vi "Sample changer.vi"() -> ()   [LabVIEW 2016, in "Top Level.lvlib"]
uses:
  Top Level.lvlib
  Sample Changer 2008 BETA 3.10.3/Visual Readback/half extended piston (push).ctl
  Sample Changer 2008 BETA 3.10.3/Visual Readback/half extended piston (push-in).ctl
  Sample Changer 2008 BETA 3.10.3/Visual Readback/Sample Rod (mid).ctl
  Sample Changer 2008 BETA 3.10.3/Visual Readback/Sample Rod (up-empty).ctl
  Sample Changer 2008 BETA 3.10.3/Visual Readback/Sample Rod (up-cathode).ctl
  Sample Changer 2008 BETA 3.10.3/Visual Readback/Sample Rod (down).ctl
  Sample Changer 2008 BETA 3.10.3/Visual Readback/Error - 2 Cathodes in the Rod.ctl
  Sample Changer 2008 BETA 3.10.3/Visual Readback/Wheel Gate Valve.ctl
panel:
  out "Wheel Gate Valve":T1
  out "Error - 2 Cathodes In Wheel":T2
  out "Error - 2 Cathodes In Rod":T2
  out "Sample Rod (down)":T3
  out "Wheel (Rod through)":bool
  out "Wheel (Empty)":bool
  out "Wheel (non-cathode position)":bool
  out "Wheel (cathode position)":bool
  out "Sample Rod (up-cathode)":T4
  out "Sample Rod (empty)":T5
  out "Sample Rod (mid)":T6
  out "half extended piston (in)":T7
  out "Extended Piston (in)":bool
  out "half extended piston (out)":T8
  out "Extended Piston (out)":bool
  in  "Encoder Home Off-Set":dbl=2790.0
  in  "sample number 2":i16
  out "Shared Network Variable Error":errorcluster
  out "Bellows Pressure String Read Error":errorcluster
  out "Source Pressure String Read Error":errorcluster
  out "output 1":dbl
  out "output 2":dbl
  in  "vent system":bool
  in  "stop":bool
  out "change sample":bool
  in  "cold cathode":dbl format="%#_3e"
  in  "Bellows pressure(torr)":string
  in  "Source pressure(torr)":string
  out "read position":dbl
  out "insert in":bool
  out "insert out":bool
  out "retract in":bool
  out "retract out":bool
  out "rod  down":bool
  out "rod up":bool
  out "sc gv closed":bool
  out "sc gv open":bool
  in  "rotate wheel":bool
  in  "sample number":i16
  in  "sc control":string
  in  "turn cold cathode off":bool
  in  "turn cold cathode on":bool
  in  "insert in":bool
  in  "insert out":bool
  in  "pump out system":bool
  in  "retract in":bool
  in  "retract out":bool
  in  "rod down":bool
  in  "rod up":bool
  in  "chamber valve close":bool
  in  "chamber valve open":bool
  # "Opens or Closes Wheel chamber valve"
  # "rotate wheel or change sample"
  # "Inserts sample into wheel"
  # "Pushes sample out of wheel"
  # "Raises or lowers Sample Rod"
  # "Turn cold cathode gauge on and off"
  # "If the cathode position is too low:\nYou have to increase the value.\nToo high, you have to lower it."
  # "vent system= isolate wheel chamber from bellows and source\nPump out system = re-connect wheel chamber to bellows and source"
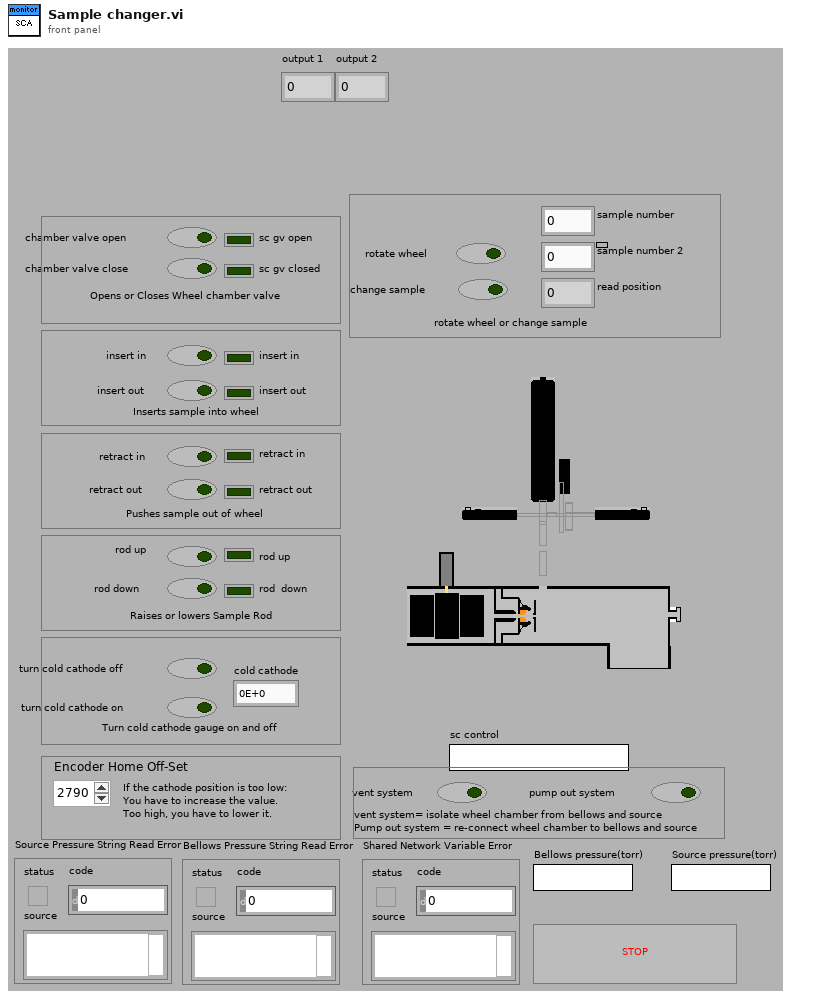
[diagram p1: front panel]
types:
  T1 = typedef "Wheel Gate Valve.ctl" = bool
  T2 = typedef "Error - 2 Cathodes in the Rod.ctl" = bool
  T3 = typedef "Sample Rod (down).ctl" = bool
  T4 = typedef "Sample Rod (up-cathode).ctl" = bool
  T5 = typedef "Sample Rod (up-empty).ctl" = bool
  T6 = typedef "Sample Rod (mid).ctl" = bool
  T7 = typedef "half extended piston (push-in).ctl" = bool
  T8 = typedef "half extended piston (push).ctl" = bool
  T9 = typedef "Device Position Enum.ctl" = enum16{"Unknown", "Actuator Is Moving", "Actuator Is Extended", "Actuator Is Retracted", "Disabled"}
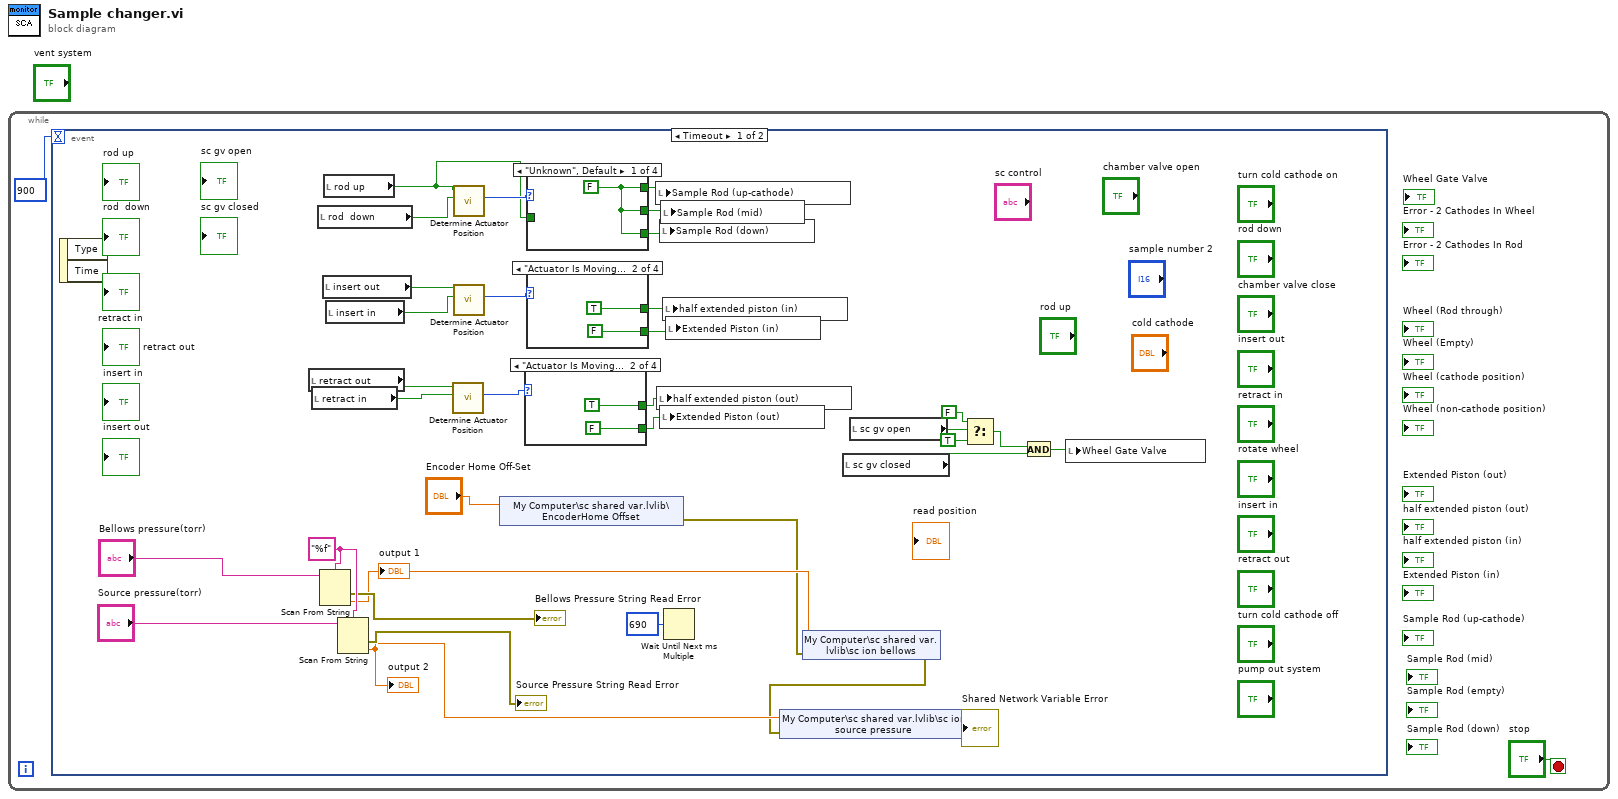
[diagram p0: block diagram]
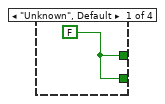
[diagram p2: hidden frame]
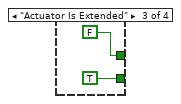
[diagram p3: hidden frame]
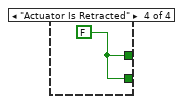
[diagram p4: hidden frame]
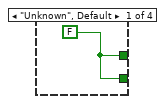
[diagram p5: hidden frame]
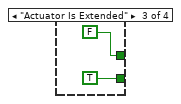
[diagram p6: hidden frame]
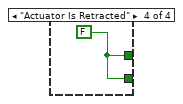
[diagram p7: hidden frame]
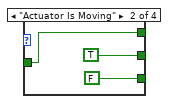
[diagram p8: hidden frame]
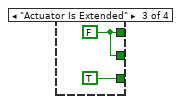
[diagram p9: hidden frame]
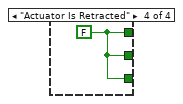
[diagram p10: hidden frame]
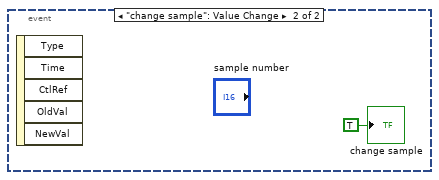
[diagram p11: hidden frame]
diagram:
  n1 = while {
    stop <- "stop" stop-if-true
    n2 = event shown="[0] Timeout" {
      selector: _ -> [_ _]
      dyn-events: _ -> [_ _]
      timeout: 900 -> [_ _]
      event Timeout {
        w35 = "%f" ("format string")
        n3 = event-data() -> ()  [unwired: 1 in, 2 out]
        n4 = local read "retract out"() -> (w5:bool)
        n5 = local read "retract in"() -> (w4:bool)
        n6 = local read "rod  down"() -> (w14:bool)
        n7 = Scan From String(format string=w35, input string="Bellows pressure(torr)") -> (error out=→"Bellows Pressure String Read Error":errorcluster, output 1=w32:dbl)  [unwired: 3 in, 2 out]
        "output 1" <- w32
        n8 = local read "insert out"() -> (w7:bool)
        n9 = local read "rod up"() -> (w3:bool)
        n10 = local read "insert in"() -> (w6:bool)
        n11 = Scan From String(format string=w35, input string="Source pressure(torr)") -> (error out=→"Source Pressure String Read Error":errorcluster, output 1=w31:dbl)  [unwired: 3 in, 2 out]
        "output 2" <- w31
        n12 = call "Determine Actuator Position.vi"("Extended Lead"=w4, "Retracted Lead"=w5) -> ("Actuator Position Enum"=w22:T9)  [unwired: 1 in, 8 out]
        n13 = call "Determine Actuator Position.vi"("Extended Lead"=w14, "Retracted Lead"=w3) -> ("Actuator Position Enum"=w24:T9)  [unwired: 1 in, 8 out]
        n14 = call "Determine Actuator Position.vi"("Extended Lead"=w6, "Retracted Lead"=w7) -> ("Actuator Position Enum"=w23:T9)  [unwired: 1 in, 8 out]
        n15 = shared-variable "My Computer\\sc shared var.lvlib\\EncoderHome Offset"("Encoder Home Off-Set") -> (error out=w25:errorcluster)  [unwired: 1 in]
        n16 = case shown="\"Actuator Is Moving\"" w22 {
          tunnel: [w37 FALSE TRUE w42] -> w16
          tunnel: [w37 TRUE FALSE ("Time Out Occured") w42] -> w15
          frame "Unknown", Default {
            w37 = FALSE ("Time Out Occured")
          }
          frame "Actuator Is Moving" {
          }
          frame "Actuator Is Extended" {
          }
          frame "Actuator Is Retracted" {
            w42 = FALSE ("Time Out Occured")
          }
        }
        n17 = case shown="\"Unknown\", Default" w24 {
          tunnel: w3 -> [_ w52 _ _]
          tunnel: [w49 FALSE TRUE w55] -> w19
          tunnel: [w49 TRUE w54 w55] -> w20
          tunnel: [w49 w52 w54 w55] -> w21
          frame "Unknown", Default {
            w49 = FALSE ("Time Out Occured")
          }
          frame "Actuator Is Moving" {
          }
          frame "Actuator Is Extended" {
            w54 = FALSE ("Time Out Occured")
          }
          frame "Actuator Is Retracted" {
            w55 = FALSE ("Time Out Occured")
          }
        }
        n18 = case shown="\"Actuator Is Moving\"" w23 {
          tunnel: [w43 FALSE TRUE w48] -> w17
          tunnel: [w43 TRUE FALSE ("Time Out Occured") w48] -> w18
          frame "Unknown", Default {
            w43 = FALSE ("Time Out Occured")
          }
          frame "Actuator Is Moving" {
          }
          frame "Actuator Is Extended" {
          }
          frame "Actuator Is Retracted" {
            w48 = FALSE ("Time Out Occured")
          }
        }
        n19 = local write "Sample Rod (up-cathode)"(w21) -> ()
        n20 = local write "half extended piston (out)"(w15) -> ()
        n21 = local write "Sample Rod (down)"(w19) -> ()
        n22 = local write "Extended Piston (out)"(w16) -> ()
        n23 = local write "Sample Rod (mid)"(w20) -> ()
        n24 = local write "half extended piston (in)"(w18) -> ()
        n25 = Wait Until Next ms Multiple(millisecond multiple=u32 690) -> ()  [unwired: 1 out]
        n26 = local write "Extended Piston (in)"(w17) -> ()
        n27 = shared-variable "My Computer\\sc shared var.lvlib\\sc ion bellows"(w32, error in=w25) -> (error out=w28:errorcluster)
        n28 = shared-variable "My Computer\\sc shared var.lvlib\\sc ion source pressure"(w31, error in=w28) -> (error out=→"Shared Network Variable Error":errorcluster)
        n29 = local read "sc gv closed"() -> (w8:bool)
        n30 = local read "sc gv open"() -> (w13:bool)
        n31 = Select(t=FALSE, s=w13, f=TRUE) -> (s? t:f=w10:bool)
        n32 = And(x=w10, y=w8) -> (x .and. y?=w9:bool)
        n33 = local write "Wheel Gate Valve"(w9) -> ()
      }
      event "change sample": Value Change {
        n34 = event-data() -> ()  [unwired: 1 in, 5 out]
        "change sample" <- TRUE ("change sample")
      }
    }
  }
